vi "Configure Front Panel Size.vi"(8 "error in":errorcluster, 11 "VI ref":refnum<vi>) -> (0 "error out":errorcluster, 1 "applied":bool)   [LabVIEW 2012, in "NI_SE_Config Front Panel Layout.lvlib"]
uses:
  NI_SE_Config Front Panel Layout.lvlib
panel:
  in  "apply":bool
  in  "Height":i32 min=0
  in  "Width":i32 min=0
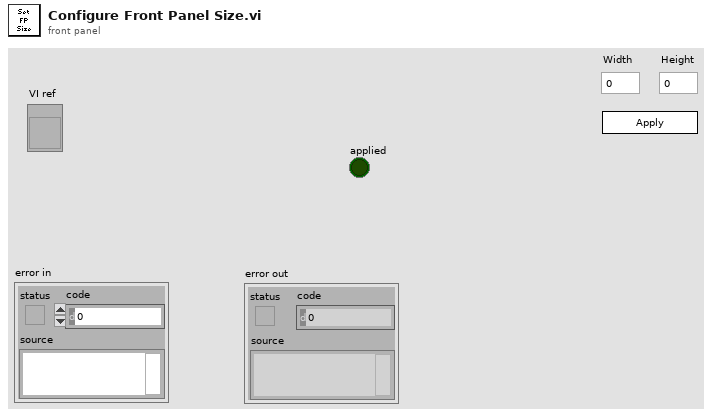
[diagram p1: front panel]
types:
  T1 = typedef "LVRectTypeDef.ctl" = cluster{"Left":i16, "Top":i16, "Right":i16, "Bottom":i16}
  T2 = typedef "LVPointTypeDef.ctl" = cluster{"Horizontal":i16, "Vertical":i16}
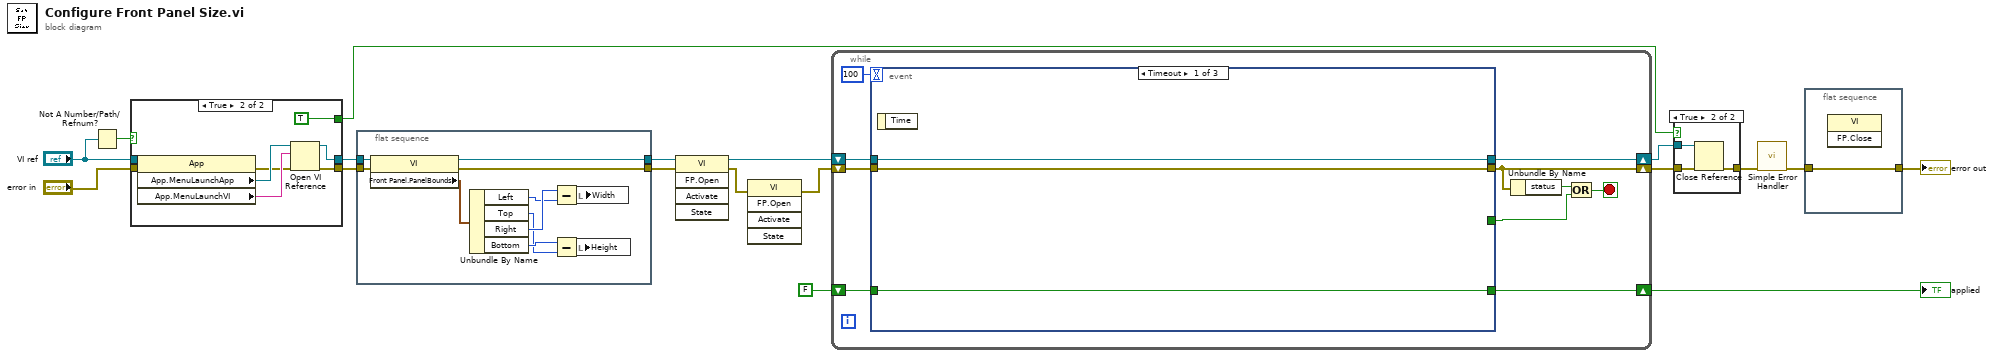
[diagram p0: block diagram]
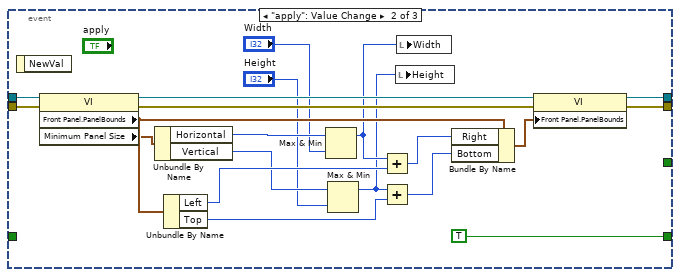
[diagram p4: hidden frame]
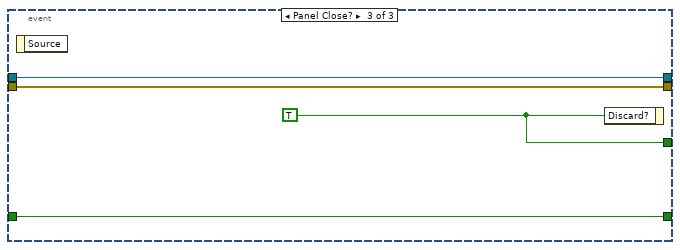
[diagram p5: hidden frame]
diagram:
  n1 = Not A Number/Path/Refnum?(number/path/refnum="VI ref") -> (NaN/Path/Refnum?=w12:bool)
  n2 = case shown="True" w12 {
    tunnel: [w20 w24] -> w16
    tunnel: [w19 w23] -> w15
    tunnel: "VI ref" -> [w20 _]
    tunnel: "error in" -> [w19 w22]
    tunnel: [_ TRUE] -> w8
    frame False {
    }
    frame True {
      n3 = property class="App"(error in=w22) -> (error out=w25:errorcluster, "App.MenuLaunchApp"=w27:refnum<vi>, "App.MenuLaunchVI"=w26:string)  [unwired: 1 in, 1 out]
      n4 = Open VI Reference(application reference (local)=w27, vi path=w26, error in (no error)=w25) -> (vi reference=w24:refnum<vi>, error out=w23:errorcluster)  [unwired: 3 in]
    }
  }
  n5 = flat-sequence {
    tunnel: w16 -> [w38]
    tunnel: [w37] -> w5
    tunnel: w15 -> [w36]
    tunnel: [w28] -> w4
    frame #0 {
      n6 = property class="VI"(reference=w38, error in=w36) -> (reference out=w37:refnum<vi>, error out=w28:errorcluster, "Front Panel.PanelBounds"=w35:T1)
      n7 = Unbundle By Name(w35) -> ("Left"=w33:i16, "Top"=w30:i16, "Right"=w34:i16, "Bottom"=w31:i16)
      n8 = Subtract(x=w34, y=w33) -> (x-y=w32:i16)
      n9 = Subtract(x=w31, y=w30) -> (x-y=w29:i16)
      n10 = local write "Height"(w29) -> ()
      n11 = local write "Width"(w32) -> ()
    }
  }
  n12 = invoke class="VI" method="FP.Open"(reference=w5, error in=w4) -> (reference out=w6:refnum<vi>, error out=w3:errorcluster)  [unwired: 3 in, 3 out]
  n13 = invoke class="VI" method="FP.Open"(error in=w3) -> (error out=w7:errorcluster)  [unwired: 4 in, 4 out]
  n14 = while {
    shift-right: [w45] -> w14
    shift-left: w7 -> [w48]
    shift-right: [w46] -> w13
    shift-left: w6 -> [w47]
    shift-right: [w39] -> w1
    shift-left: FALSE -> [w40]
    stop <- w42 stop-if-true
    n15 = event shown="[0] Timeout" {
      selector: _ -> [_ _ _]
      dyn-events: _ -> [_ _ _]
      timeout: 100 -> [_ _ _]
      tunnel: w48 -> [w50 w70 w75]
      tunnel: w47 -> [w51 w71 w74]
      tunnel: [w50 w65 w75] -> w45
      tunnel: [w51 w64 w74] -> w46
      tunnel: [_ _ w73] -> w43
      tunnel: w40 -> [w49 _ w72]
      tunnel: [w49 TRUE w72] -> w39
      event Timeout {
        n16 = event-data() -> ()  [unwired: 1 in, 1 out]
      }
      event "apply": Value Change {
        n17 = event-data() -> ()  [unwired: 1 in, 1 out]
        n18 = property class="VI"(reference=w71, error in=w70) -> (reference out=w67:refnum<vi>, error out=w66:errorcluster, "Front Panel.PanelBounds"=w69:T1, "Minimum Panel Size"=w63:T2)
        n19 = Unbundle By Name(w63) -> ("Horizontal"=w62:i16, "Vertical"=w59:i16)
        n20 = Unbundle By Name(w69) -> ("Left"=w61:i16, "Top"=w54:i16)
        n21 = Max & Min(x=w62, y="Width") -> (max(x,y)=w55:i32)  [unwired: 1 out]
        n22 = Max & Min(x=w59, y="Height") -> (max(x,y)=w53:i32)  [unwired: 1 out]
        n23 = Add(x=w55, y=w61) -> (x+y=w60:i32)
        n24 = Add(x=w53, y=w54) -> (x+y=w58:i32)
        n25 = local write "Height"(w53) -> ()
        n26 = local write "Width"(w55) -> ()
        n27 = Bundle By Name(cluster=w69, "Right"=w60, "Bottom"=w58) -> (w68:T1)
        n28 = property class="VI"(reference=w67, error in=w66, "Front Panel.PanelBounds"=w68) -> (reference out=w64:refnum<vi>, error out=w65:errorcluster)
      }
      event Panel Close? {
        w73 = TRUE ("Discard?")
        n29 = event-data() -> ()  [unwired: 1 in, 1 out]
        n30 = event-data("Discard?"=w73) -> ()  [unwired: 1 in, 1 out]
      }
    }
    n31 = Unbundle By Name(w45) -> ("status"=w44:bool)
    n32 = Or(x=w44, y=w43) -> (x .or. y?=w42:bool)
  }
  "applied" <- w1
  n33 = case shown="True" w8 {
    tunnel: [w76 w79] -> w17
    tunnel: w14 -> [w76 w78]
    tunnel: w13 -> [_ w77]
    frame False {
    }
    frame True {
      n34 = Close Reference(reference=w77, error in (no error)=w78) -> (error out=w79:errorcluster)
    }
  }
  n35 = call <vilib>:"Simple Error Handler.vi"("error in (no error)"=w17) -> ("error out"=w18:errorcluster)  [unwired: 4 in, 4 out]
  n36 = flat-sequence {
    tunnel: w18 -> [w80]
    tunnel: [w80] -> w9
    frame #0 {
      n37 = invoke class="VI" method="FP.Close"() -> ()  [unwired: 3 in, 3 out]
    }
  }
  "error out" <- w9
